vi "PR_Update_Workspace .vi"(7 "[workplace_id]":i16=2, 8 "error in (no error)":errorcluster, 10 "barcode":string="123465798", 11 "DBlink":string="Driver={ODBC Driver 17 for SQL Server};Server=localhost\\SQLEXPRESS;Database=ZDX201;UID=labview;PWD=Dsa@54137926") -> (0 "error out":errorcluster)   [LabVIEW 2019]
uses:
  <vilib>/addons/database/Connection.llb/DB Tools Open Connec (String).vi
  <vilib>/addons/database/NI_Database_API.lvlib
panel:
  out "concatenated string":string="WHERE [barcode]='123465798' and [pos]='A'"
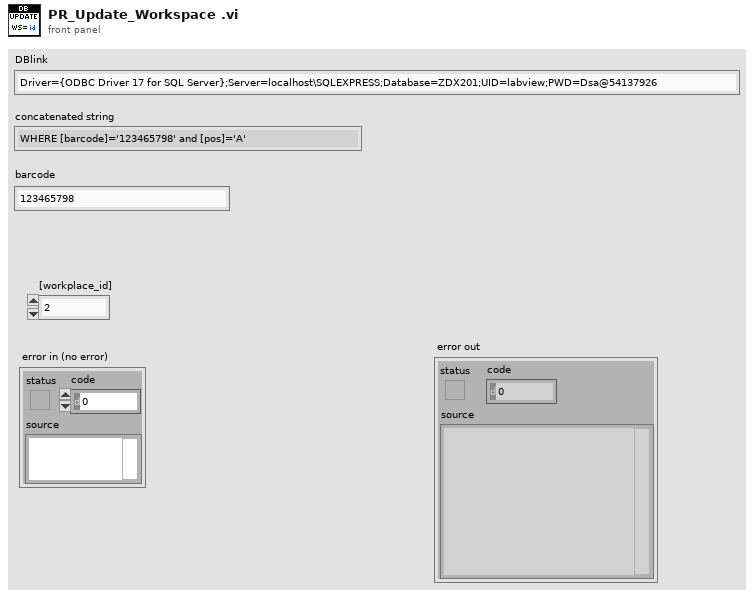
[diagram p1: front panel]
types:
  T1 = cluster{"[workplace_id]":i16, "update_time":timestamp}
  T2 = typedef "NI_Database_API.lvlib/Conn ObjectReference.ctl" = refnum<k1>
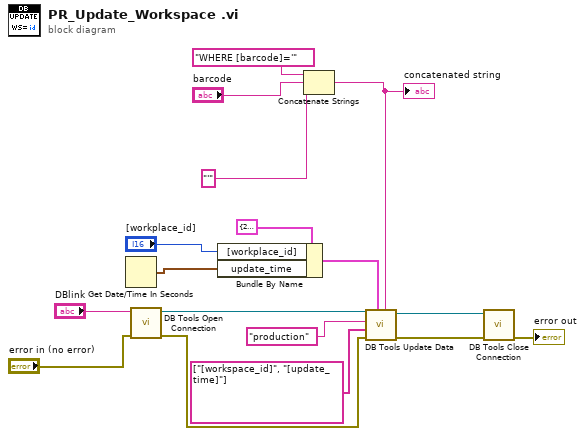
[diagram p0: block diagram]
diagram:
  n1 = Get Date/Time In Seconds() -> (seconds since 1Jan1904=w2:timestamp)
  n2 = call-poly <vilib>:"DB Tools Open Connection.vi"("error in (no error)"="error in (no error)", "connection information"="DBlink") -> ("error out"=w15:errorcluster, "connection reference"=w13:T2)  [unwired: 6 in]
  n3 = Bundle By Name(cluster=T1 {"[workplace_id]"=2, "update_time"=timestamp(0 s since 1904-01-01)}, "[workplace_id]"="[workplace_id]", "update_time"=w2) -> (w1:T1)
  n4 = Concatenate Strings("WHERE [barcode]='", "barcode", "'" ("string")) -> (w7:string)
  "concatenated string" <- w7
  n5 = call <vilib>:"DB Tools Update Data.vi"("condition"=w7, "data"=w1, "error in (no error)"=w15, "columns"=string[] ["[workspace_id]", "[update_time]"], "table"="production", "connection reference"=w13) -> ("error out"=w16:errorcluster, "connection reference out"=w14:T2)  [unwired: 4 in]
  n6 = call <vilib>:"DB Tools Close Connection.vi"("error in (no error)"=w16, "connection reference"=w14) -> ("error out"=→"error out":errorcluster)  [unwired: 5 in]
